vi "PullValuesFromControls.vi"(8 "error in (no error)":errorcluster, 10 "ControlNameArray":string[](array[string]), 11 "Variant In":variant) -> (0 "error out":errorcluster, 2 "ControlValuesArray":sgl[](array[numeric]), 3 "Variant out":variant)   [LabVIEW 2016, in "M1M3SupportEUI_Views.lvlib"]
uses:
  M1M3SupportEUI_Views.lvlib
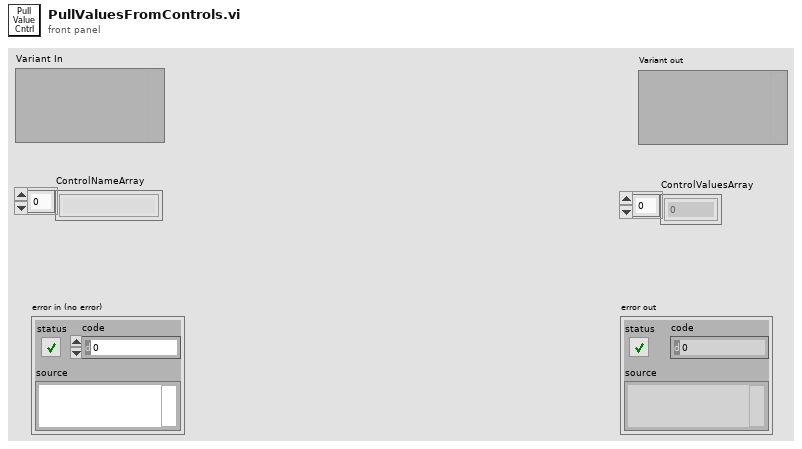
[diagram p1: front panel]
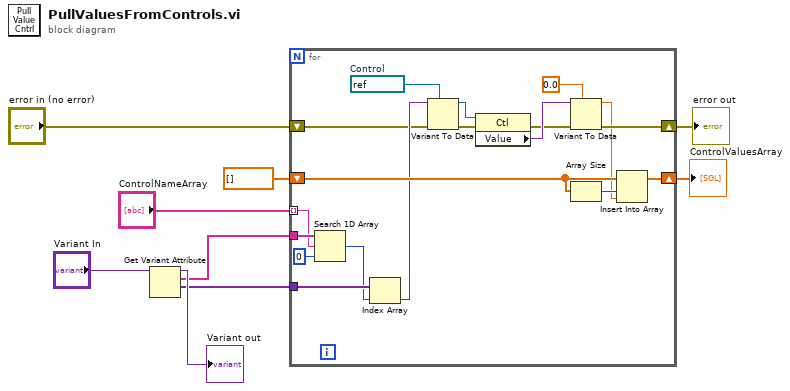
[diagram p0: block diagram]
diagram:
  n1 = Get Variant Attribute(Variant="Variant In") -> (duplicate Variant=→"Variant out":variant, names=w2:string[], values=w1:variant[])  [unwired: 3 in, 1 out]
  n2 = for {
    tunnel: "ControlNameArray" -> [w15] mode=indexing
    shift-right: [w27] -> w8
    shift-left: sgl[] [] -> [w25]
    shift-right: [w19] -> w5
    shift-left: "error in (no error)" -> [w10]
    tunnel: w2 -> [w16]
    tunnel: w1 -> [w14]
    w24 = refnum<vi> refnum  # Control
    n3 = Search 1D Array(1D array=w16, element=w15, start index (0)=0) -> (index of element=w13:i32)
    n4 = Index Array(array=w14, index=w13) -> (element=w11:variant)
    n5 = Variant To Data(error in=w10, type=w24, Variant=w11) -> (data=w23:refnum<vi>, error out=w22:errorcluster)
    n6 = property class="Ctl"(reference=w23, error in=w22) -> (error out=w20:errorcluster, "Value"=w21:variant)  [unwired: 1 out]
    n7 = Variant To Data(error in=w20, type=sgl 0.0, Variant=w21) -> (data=w17:sgl, error out=w19:errorcluster)
    n8 = Array Size(array=w25) -> (size(s)=w26:i32)
    n9 = Insert Into Array(array=w25, index=w26, new element=w17) -> (w27:sgl[])
  }
  "error out" <- w5
  "ControlValuesArray" <- w8
